vi "Save.vi"(8 "error in (no error)":errorcluster, 9 "new command":string, 10 "Msg in":T1, 11 "FakePressureController in":refnum<class "MagAnalysis_Online.lvclass">) -> (0 "error out":errorcluster, 1 "Path":path, 2 "Msg out":T1, 3 "FakePressureController out":refnum<class "MagAnalysis_Online.lvclass">, 4 "new command":string)   [LabVIEW 2013, in "MagAnalysis_Online.lvclass"]
uses:
  MagAnalysis_Online.lvclass
  BaseDriver/DriverMsg.ctl
  MagAnalysis_Online.lvclass/MagAnalysis_Online.ctl
  DaqPad_NI6009/DaqPad_NI6009.lvclass
panel:
  out "error out 2":errorcluster
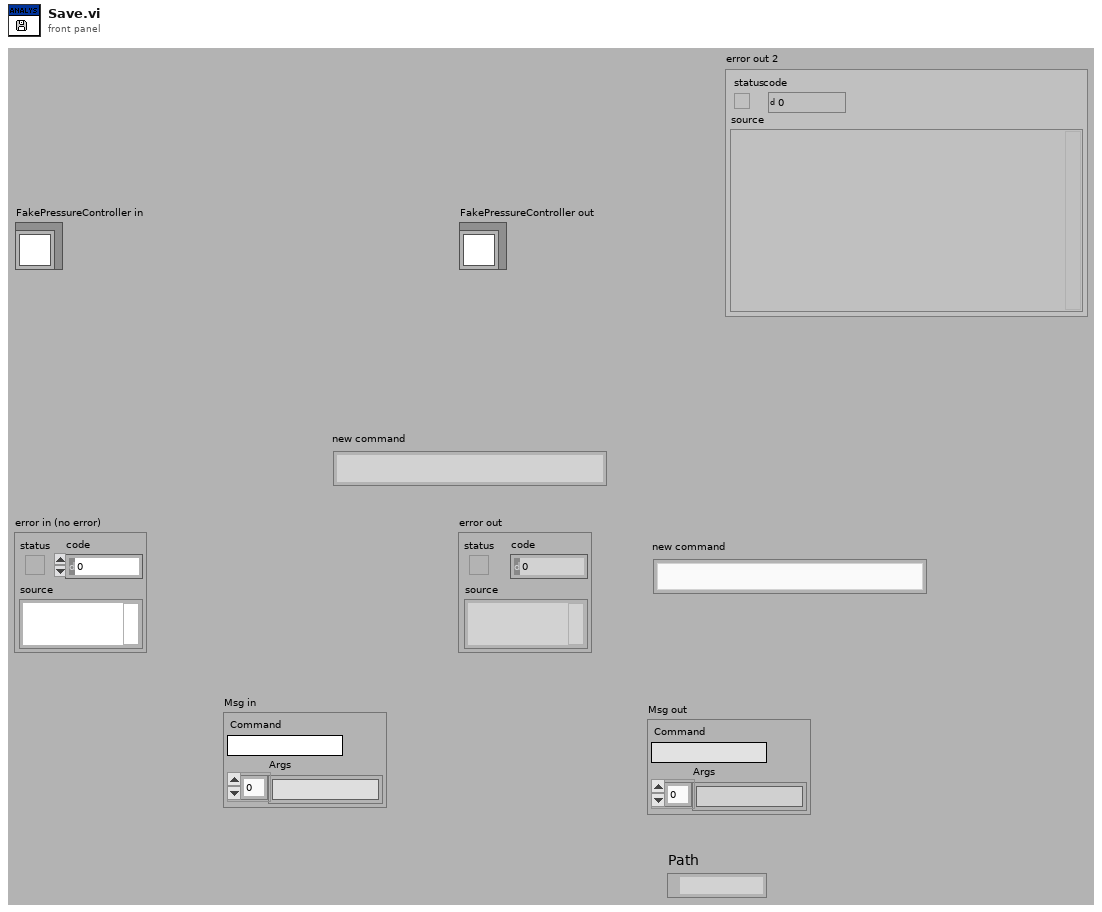
[diagram p1: front panel]
types:
  T1 = typedef "DriverMsg.ctl" = cluster{"Command":string, "Args":string[]}
  T2 = typedef "IMAQ Image.ctl" = refnum<image>
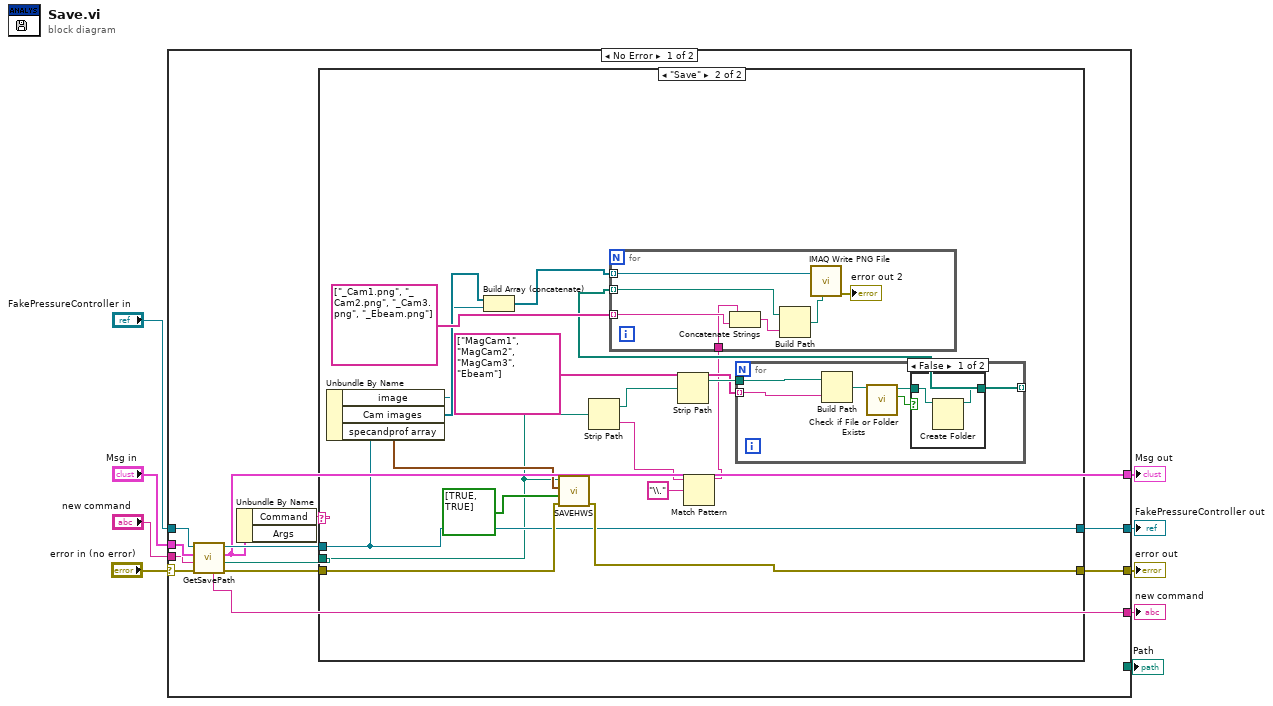
[diagram p0: block diagram]
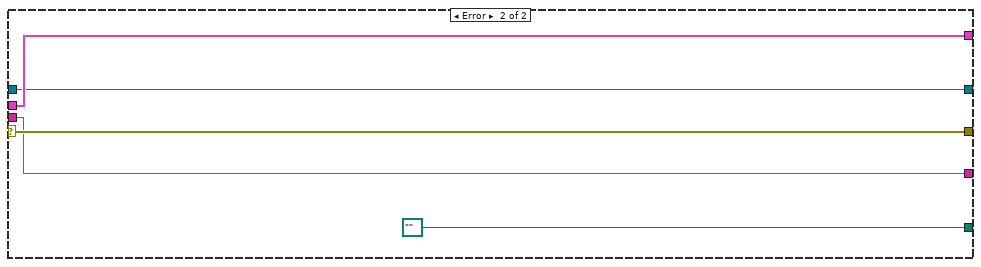
[diagram p4: hidden frame]
diagram:
  n1 = case shown="No Error" "error in (no error)" {
    selector: "error in (no error)" -> [w15 w61]
    tunnel: [w19 w61] -> w5
    tunnel: [_ path "" ("Path")] -> w1
    tunnel: [w13 w60] -> w6
    tunnel: [w20 w59] -> w8
    tunnel: "Msg in" -> [w17 w60]
    tunnel: "FakePressureController in" -> [w18 w59]
    tunnel: "new command" -> [w16 w57]
    tunnel: [w10 w57] -> w2
    frame No Error {
      n2 = call-dynamic "GetSavePath.vi"("error in (no error)"=w15, "new command"=w16, "Msg in"=w17, "BaseDriver in"=w18) -> ("error out"=w11:errorcluster, "Path"=w12:path, "Msg out"=w13:T1, "BaseDriver out"=w14:refnum<class "MagAnalysis_Online.lvclass">, "new command"=w10:string)  [unwired: 3 in]
      n3 = Unbundle By Name(w13) -> ("Command"=w21:string)  [unwired: 1 out]
      n4 = case shown="\"Save\"" w21 {
        tunnel: w14 -> [w23 w37]
        tunnel: [w23 w37] -> w20
        tunnel: w12 -> [_ w35]
        tunnel: w11 -> [w22 w39]
        tunnel: [w22 w38] -> w19
        frame Default {
        }
        frame "Save" {
          n5 = Unbundle By Name(w37) -> ("image"=w25:T2, "Cam images"=w26:T2[], "specandprof array"=w36:waveform(dbl)[])
          n6 = Build Array (concatenate)(w26, w25) -> (w24:T2[])
          n7 = call "SAVEHWS.vi"("error in (no error)"=w39, "Enable (Array)"=bool[] [TRUE, TRUE], "data"=w36, "Destination HWS File"=w35) -> ("error out"=w38:errorcluster)  [unwired: 7 in]
          n8 = Strip Path(path=w35) -> (stripped path=w27:path, name=w33:string)
          n9 = Strip Path(path=w27) -> (stripped path=w31:path)  [unwired: 1 out]
          n10 = Match Pattern(string=w33, regular expression="\\.") -> (before substring=w28:string)  [unwired: 1 in, 3 out]
          n11 = for {
            tunnel: w31 -> [w46]
            tunnel: string[] ["MagCam1", "MagCam2", "MagCam3", "Ebeam"] -> [w45] mode=indexing
            tunnel: [w41] -> w29 mode=indexing
            n12 = Build Path(base path=w46, name or relative path=w45) -> (appended path=w44:path)
            n13 = call <vilib>:"Check if File or Folder Exists.vi"("path"=w44) -> ("file or folder exists?"=w42:bool, "dup path"=w43:path)  [unwired: 8 in, 1 out]
            n14 = case shown="False" w42 {
              tunnel: w43 -> [w48 w49]
              tunnel: [w47 w49] -> w41
              frame False {
                n15 = Create Folder(path (use dialog)=w48) -> (created path=w47:path)  [unwired: 2 in, 2 out]
              }
              frame True {
              }
            }
          }
          n16 = for {
            tunnel: w29 -> [w53] mode=indexing
            tunnel: string[] ["_Cam1.png", "_Cam2.png", "_Cam3.png", "_Ebeam.png"] -> [w52] mode=indexing
            tunnel: w24 -> [w51] mode=indexing
            tunnel: w28 -> [w50]
            n17 = Concatenate Strings(w50, w52) -> (w54:string)
            n18 = Build Path(base path=w53, name or relative path=w54) -> (appended path=w55:path)
            n19 = call "IMAQ Write PNG File"("File Path"=w55, "Image"=w51) -> ("error out"=→"error out 2":errorcluster)  [unwired: 4 in, 2 out]
          }
        }
      }
    }
    frame Error {
    }
  }
  "error out" <- w5
  "FakePressureController out" <- w8
  "Path" <- w1
  "Msg out" <- w6
  "new command" <- w2
